vi "Gen - Check for Active Page.vi"(8 "Error In":errorcluster, 10 "VI Name in":string, 11 "This VI":refnum<vi>) -> (0 "Error Out":errorcluster, 2 "This VI Name":string, 3 "Active Page?":bool)   [LabVIEW 2020]
doc: "This VI use to get VI name. This VI name normally use to compare with active page."
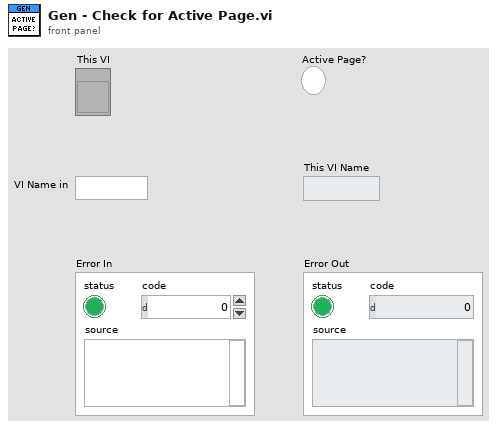
[diagram p1: front panel]
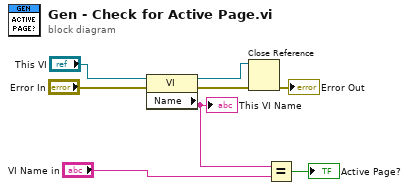
[diagram p0: block diagram]
diagram:
  n1 = property class="VI"(reference="This VI", error in="Error In") -> (reference out=w5:refnum<vi>, error out=w8:errorcluster, "Name"=w3:string)
  "This VI Name" <- w3
  n2 = Close Reference(reference=w5, error in (no error)=w8) -> (error out=→"Error Out":errorcluster)
  n3 = Equal?(x=w3, y="VI Name in") -> (x = y?=→"Active Page?":bool)
